vi "Destroy DebugTerminal.vi"(8 "error in (no error)":errorcluster, 11 "DebuggingTerminal in":refnum<class "DebuggingTerminal.lvclass">) -> (0 "error out":errorcluster, 3 "DebuggingTerminal out":refnum<class "DebuggingTerminal.lvclass">)   [LabVIEW 2013, in "MQTT Base.lvlib" / "DebuggingTerminal.lvclass"]
uses:
  DebuggingTerminal.lvclass
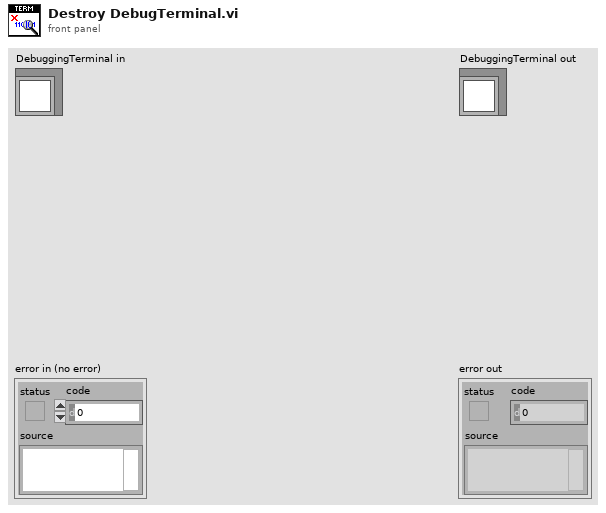
[diagram p1: front panel]
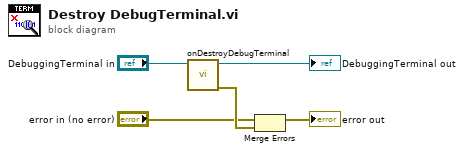
[diagram p0: block diagram]
diagram:
  n1 = call-dynamic "onDestroyDebugTerminal.vi"("DebuggingTerminal in"="DebuggingTerminal in") -> ("error out"=w3:errorcluster, "DebuggingTerminal out"=→"DebuggingTerminal out":refnum<class "DebuggingTerminal.lvclass">)  [unwired: 9 in]
  n2 = Merge Errors("error in (no error)", w3) -> (→"error out":errorcluster)
